vi "HFRR ADV v03.vi"() -> ()   [LabVIEW 2025] (continued)
                  n2418 = local write "S 85"(w3547) -> ()
                }
                frame 84 {
                  n2419 = local write "S 86"(w3548) -> ()
                }
                frame 85 {
                  n2420 = local write "S 87"(w3549) -> ()
                }
                frame 86 {
                  n2421 = local write "S 88"(w3550) -> ()
                }
                frame 87 {
                  n2422 = property on="FF Calibration g" class="WFGraph (strict)"("Y Scale.Name Label.Text"=w3551) -> ()  [unwired: 2 in, 2 out]
                }
                frame 88 {
                  n2423 = local write "S 90"(w3552) -> ()
                }
                frame 89 {
                  n2424 = local write "S 91"(w3553) -> ()
                }
                frame 90 {
                  n2425 = local write "S 92"(w3554) -> ()
                }
                frame 91 {
                  n2426 = local write "S 93"(w3555) -> ()
                }
                frame 92 {
                  n2427 = local write "S 94"(w3556) -> ()
                }
                frame 93 {
                  n2428 = local write "S 95"(w3557) -> ()
                }
                frame 94 {
                  n2429 = local write "S 96"(w3558) -> ()
                }
                frame 95 {
                  n2430 = local write "S 97"(w3559) -> ()
                }
                frame 96 {
                  n2431 = local write "S 98"(w3560) -> ()
                }
                frame 97 {
                  n2432 = local write "S 99"(w3561) -> ()
                }
                frame 98 {
                  n2433 = local write "S 100"(w3562) -> ()
                }
                frame 99 {
                  n2434 = local write "S 101"(w3563) -> ()
                }
                frame 100 {
                  n2435 = local write "S 102"(w3564) -> ()
                }
                frame 101 {
                  n2436 = local write "S 103"(w3565) -> ()
                }
                frame 102 {
                  n2437 = local write "S 104"(w3566) -> ()
                }
                frame 103 {
                  n2438 = local write "S 105"(w3567) -> ()
                }
                frame 104 {
                  n2439 = local write "S 106"(w3568) -> ()
                }
                frame 105 {
                }
                frame 106 {
                  n2440 = property on="OK Button 17" class="Bool (strict)"("Boolean Text.Text"=w3569) -> ()  [unwired: 2 in, 2 out]
                }
                frame 107 {
                  n2441 = property on="OK Button 16" class="Bool (strict)"("Boolean Text.Text"=w3570) -> ()  [unwired: 2 in, 2 out]
                }
                frame 108 {
                  n2442 = property on="TITTLE" class="Str"("Caption.Text"=w3571) -> ()  [unwired: 2 in, 2 out]
                }
                frame 109 {
                  "String 30" <- w3572
                }
                frame 110 {
                  n2443 = property on="Test Date" class="Str"("Caption.Text"=w3573) -> ()  [unwired: 2 in, 2 out]
                  "String 31" <- w3573
                }
                frame 111 {
                  n2444 = property on="Sample ID" class="Str"("Caption.Text"=w3574) -> ()  [unwired: 2 in, 2 out]
                  "String 32" <- w3574
                }
                frame 112 {
                  n2445 = property on="Tested by" class="Str"("Caption.Text"=w3575) -> ()  [unwired: 2 in, 2 out]
                  "String 33" <- w3575
                }
                frame 113 {
                  n2446 = property on="System Configured Printers 2" class="Arr (strict)"("Caption.Text"=w3576) -> ()  [unwired: 2 in, 2 out]
                }
                frame 114 {
                  n2447 = property on="Selected Printer" class="Str"("Caption.Text"=w3577) -> ()  [unwired: 2 in, 2 out]
                }
                frame 115 {
                  n2448 = property on="Select Printer 3" class="DigNum (strict)"("Caption.Text"=w3578) -> ()  [unwired: 2 in, 2 out]
                }
                frame 116 {
                  n2449 = property on="Print" class="Bool (strict)"("Boolean Text.Text"=w3579) -> ()  [unwired: 2 in, 2 out]
                }
                frame 117 {
                  "String 41" <- w3580
                }
                frame 118 {
                  n2450 = property on="tested by" class="Str"("Caption.Text"=w3581) -> ()  [unwired: 2 in, 2 out]
                }
                frame 119 {
                }
                frame 120 {
                  n2451 = property on="Export" class="Bool (strict)"("Boolean Text.Text"=w3582) -> ()  [unwired: 2 in, 2 out]
                }
                frame 121 {
                  n2452 = property on="TEMP INTERCEPT:" class="DigNum (strict)"("Caption.Text"=w3583) -> ()  [unwired: 2 in, 2 out]
                }
                frame 122 {
                  n2453 = property on="AIR TEMP INTERCEPT:" class="DigNum (strict)"("Caption.Text"=w3584) -> ()  [unwired: 2 in, 2 out]
                }
                frame 123 {
                  n2454 = property on="Select File Type" class="Enum (strict)"("Caption.Text"=w3585) -> ()  [unwired: 2 in, 2 out]
                }
                frame 124 {
                  n2455 = property on="s.NO" class="Str"("Caption.Text"=w3586) -> ()  [unwired: 2 in, 2 out]
                  "String 45" <- w3586
                }
                frame 125 {
                  n2456 = property on="trip1 8" class="Bool (strict)"("Boolean Text.Text"=w3587) -> ()  [unwired: 2 in, 2 out]
                }
                frame 126, Default {
                }
              }
            }
          }
          frame #1 {
            w3595 = TRUE ("Visible")
            n2457 = local read "S 91"() -> (w3612:string)
            n2458 = local read "S 90"() -> (w3611:string)
            n2459 = local read "S 88"() -> (w3610:string)
            n2460 = property on="Threshold" class="DigNum (strict)"("Caption.Text"=w3612) -> ()  [unwired: 2 in, 2 out]
            n2461 = property on="File Path" class="Path"("Caption.Text"=w3611) -> ()  [unwired: 2 in, 2 out]
            n2462 = property on="SrvM CP" class="Bool (strict)"("Boolean Text.Text"=w3610) -> ()  [unwired: 2 in, 2 out]
            n2463 = local read "S 71"() -> (w3605:string)
            n2464 = local read "S 86"() -> (w3607:string)
            n2465 = local read "S 85"() -> (w3608:string)
            n2466 = local read "S 87"() -> (w3606:string)
            n2467 = local read "S 84"() -> (w3609:string)
            n2468 = local read "S 103"() -> (w3594:string)
            n2469 = local read "S 104"() -> (w3593:string)
            n2470 = property on="ENTER THE NEW PASSWORD" class="Str"("Caption.Text"=w3606) -> ()  [unwired: 2 in, 2 out]
            n2471 = property on="Password" class="Str"("Caption.Text"=w3608) -> ()  [unwired: 2 in, 2 out]
            n2472 = property on="ENTER CURRENT PASSWORD" class="Str"("Caption.Text"=w3607) -> ()  [unwired: 2 in, 2 out]
            n2473 = property on="EDIT" class="Bool (strict)"("Boolean Text.Text"=w3605) -> ()  [unwired: 2 in, 2 out]
            n2474 = property on="SAVE" class="Bool (strict)"("Boolean Text.Text"=w3609) -> ()  [unwired: 2 in, 2 out]
            n2475 = Build Array(w3594, w3593) -> (w3592:string[])
            n2476 = property on="Heater Button" class="Bool (strict)"("Strings [4]"=w3592) -> ()  [unwired: 2 in, 2 out]
            n2477 = property on="CH-HUMIDITY WET" class="DigNum (strict)"("Caption.Size to Text?"=w3595) -> ()  [unwired: 2 in, 2 out]
            n2478 = property on="CH-HUMIDITY DRY" class="DigNum (strict)"("Caption.Size to Text?"=w3595) -> ()  [unwired: 2 in, 2 out]
            n2479 = property on="CH-POWER -" class="DigNum (strict)"("Caption.Size to Text?"=w3595) -> ()  [unwired: 2 in, 2 out]
            n2480 = property on="CH-HEATER" class="DigNum (strict)"("Caption.Size to Text?"=w3595) -> ()  [unwired: 2 in, 2 out]
            n2481 = property on="CH-POWER +" class="DigNum (strict)"("Caption.Size to Text?"=w3595) -> ()  [unwired: 2 in, 2 out]
            n2482 = local read "S 92"() -> (w3604:string)
            n2483 = local read "S 93"() -> (w3603:string)
            n2484 = local read "S 105"() -> (w3590:string)
            n2485 = local read "S 106"() -> (w3589:string)
            n2486 = Build Array(w3604, w3603) -> ()  [unwired: 1 out]
            n2487 = Build Array(w3590, w3589) -> (w3591:string[])
            n2488 = local read "S 95"() -> (w3601:string)
            n2489 = local read "S 94"() -> (w3602:string)
            n2490 = local read "bs"() -> (w3617:string)
            n2491 = local read "as"() -> (w3618:string)
            n2492 = property on="Humidity" class="Bool (strict)"("Strings [4]"=w3591) -> ()  [unwired: 2 in, 2 out]
            n2493 = Concatenate Strings(w3617, "\r", w3618) -> ()  [unwired: 1 out]
            n2494 = property on="STROKE GAIN :" class="DigNum (strict)"("Caption.Text"=w3601) -> ()  [unwired: 2 in, 2 out]
            n2495 = property on="DISPLACEMENT :" class="DigNum (strict)"("Caption.Text"=w3602) -> ()  [unwired: 2 in, 2 out]
            n2496 = property on="Rh After" class="DigNum (strict)"("Caption.Size to Text?"=TRUE ("Caption.Size to Text")) -> ()  [unwired: 2 in, 2 out]
            n2497 = local read "S 48"() -> (w3641:string)
            n2498 = local read "S 50"() -> (w3639:string)
            n2499 = local read "S 51"() -> (w3638:string)
            n2500 = local read "S 49"() -> (w3640:string)
            n2501 = local read "S 52"() -> (w3637:string)
            n2502 = local read "as"() -> (w3622:string)
            n2503 = local read "bs"() -> (w3623:string)
            n2504 = local read "S 56"() -> (w3636:string)
            n2505 = local read "S 57"() -> (w3635:string)
            n2506 = local read "S 58"() -> (w3634:string)
            n2507 = local read "S 59"() -> (w3633:string)
            n2508 = property on="OPEN" class="Bool (strict)"("Boolean Text.Text"=w3637) -> ()  [unwired: 2 in, 2 out]
            n2509 = property on="OPEN 1" class="Bool (strict)"("Boolean Text.Text"=w3641) -> ()  [unwired: 2 in, 2 out]
            n2510 = property on="OPEN 2" class="Bool (strict)"("Boolean Text.Text"=w3640) -> ()  [unwired: 2 in, 2 out]
            n2511 = property on="OPEN 3" class="Bool (strict)"("Boolean Text.Text"=w3639) -> ()  [unwired: 2 in, 2 out]
            n2512 = property on="OPEN 4" class="Bool (strict)"("Boolean Text.Text"=w3638) -> ()  [unwired: 2 in, 2 out]
            n2513 = Concatenate Strings(w3623, "\r", w3622) -> ()  [unwired: 1 out]
            n2514 = local read "S 102"() -> (w3596:string)
            n2515 = property on="КОФ1" class="DigNum (strict)"("Caption.Text"=w3636) -> ()  [unwired: 2 in, 2 out]
            n2516 = local read "S 98"() -> (w3600:string)
            n2517 = local read "S 99"() -> (w3599:string)
            n2518 = local read "S 100"() -> (w3598:string)
            n2519 = local read "S 101"() -> (w3597:string)
            n2520 = property on="КОФ2" class="DigNum (strict)"("Caption.Text"=w3635) -> ()  [unwired: 2 in, 2 out]
            n2521 = property on="КОФ3" class="DigNum (strict)"("Caption.Text"=w3634) -> ()  [unwired: 2 in, 2 out]
            n2522 = property on="КОФ4" class="DigNum (strict)"("Caption.Text"=w3633) -> ()  [unwired: 2 in, 2 out]
            n2523 = local read "bs"() -> (w3621:string)
            n2524 = local read "as"() -> (w3620:string)
            n2525 = property on="CH-POWER +" class="DigNum (strict)"("Caption.Text"=w3600) -> ()  [unwired: 2 in, 2 out]
            n2526 = property on="CH-POWER -" class="DigNum (strict)"("Caption.Text"=w3599) -> ()  [unwired: 2 in, 2 out]
            n2527 = property on="CH-HEATER" class="DigNum (strict)"("Caption.Text"=w3598) -> ()  [unwired: 2 in, 2 out]
            n2528 = property on="CH-HUMIDITY DRY" class="DigNum (strict)"("Caption.Text"=w3597) -> ()  [unwired: 2 in, 2 out]
            n2529 = property on="CH-HUMIDITY WET" class="DigNum (strict)"("Caption.Text"=w3596) -> ()  [unwired: 2 in, 2 out]
            n2530 = local read "S 60"() -> (w3632:string)
            n2531 = local read "S 54"() -> (w3642:string)
            n2532 = Concatenate Strings(w3621, "\r", w3620) -> ()  [unwired: 1 out]
            n2533 = Concatenate Strings(w3642, w3632) -> ()  [unwired: 1 out]
            n2534 = local read "S 77"() -> (→"String 43":string)
            n2535 = local read "S 76"() -> (w3615:string)
            n2536 = local read "S 78"() -> (w3614:string)
            n2537 = local read "S 71"() -> (w3626:string)
            n2538 = local read "S 66"() -> (w3631:string)
            n2539 = local read "S 67"() -> (w3630:string)
            n2540 = local read "S 68"() -> (w3629:string)
            n2541 = local read "S 69"() -> (w3628:string)
            n2542 = local read "S 70"() -> (w3627:string)
            n2543 = property on="AIR TEMP" class="DigNum (strict)"("Caption.Text"=w3614) -> ()  [unwired: 2 in, 2 out]
            n2544 = property on="Set Strk" class="DigNum (strict)"("Caption.Text"=w3615) -> ()  [unwired: 2 in, 2 out]
            n2545 = property on="FRIC. FORCE :" class="DigNum (strict)"("Caption.Text"=w3631) -> ()  [unwired: 2 in, 2 out]
            n2546 = property on="TEMPERATURE :" class="DigNum (strict)"("Caption.Text"=w3630) -> ()  [unwired: 2 in, 2 out]
            n2547 = property on="SPEED OUT:" class="DigNum (strict)"("Caption.Text"=w3629) -> ()  [unwired: 2 in, 2 out]
            n2548 = property on="AIR TEMPERATURE :" class="DigNum (strict)"("Caption.Text"=w3628) -> ()  [unwired: 2 in, 2 out]
            n2549 = property on="HUMIDITY:" class="DigNum (strict)"("Caption.Text"=w3627) -> ()  [unwired: 2 in, 2 out]
            n2550 = property on="EDIT" class="Bool (strict)"("Boolean Text.Text"=w3626) -> ()  [unwired: 2 in, 2 out]
            n2551 = local read "S 79"() -> (w3613:string)
            n2552 = property on="Stroke" class="DigNum (strict)"("Caption.Text"=w3613) -> ()  [unwired: 2 in, 2 out]
          }
          frame #2 {
          }
        }
        n2553 = local write "Lan flag"(10.0 ("Lan flag")) -> ()
      }
    }
    n2554 = Wait (ms)(milliseconds to wait=u32 50) -> ()  [unwired: 1 out]
    n2555 = local read "EXIT"() -> (w3418:bool)
  }
  n2556 = flat-sequence {
    tunnel: w50 -> [_]
    frame #0 {
    }
    frame #1 {
      n2557 = Quit LabVIEW(quit? (T)=TRUE) -> ()
      n2558 = local write "EXIT"(FALSE ("EXIT")) -> ()
    }
  }
  n2559 = while {
    tunnel: [w3652] -> w48
    i -> [w3651]
    stop <- w3652 stop-if-true
    n2560 = local read "EXIT"() -> (w3652:bool)
    n2561 = Equal To 0?(x=w3651) -> (x = 0?=w3649:bool)
    n2562 = call "Elapsed Time3"("Time Target (s)"=45.0, "Auto Reset"=TRUE) -> ("Time has Elapsed"=w3648:bool)  [unwired: 10 in, 7 out]
    n2563 = Wait (ms)(milliseconds to wait=u32 50) -> ()  [unwired: 1 out]
    n2564 = Or(x=w3648, y=w3649) -> (x .or. y?=w3650:bool)
    n2565 = case shown="True" w3650 {
      frame False {
      }
      frame True {
        n2566 = call <vilib>:"System Exec.vi"("run minimized? (F)"=TRUE, "error in (no error)"="error in (no error)", "command line"="powercfg.exe -change -monitor-timeout-ac 0") -> ("error out"=w3663:errorcluster)  [unwired: 5 in, 3 out]
        n2567 = call <vilib>:"System Exec.vi"("run minimized? (F)"=TRUE, "error in (no error)"=w3663, "command line"="powercfg.exe -change -disk-timeout-ac 0") -> ("error out"=w3662:errorcluster)  [unwired: 5 in, 3 out]
        n2568 = call <vilib>:"System Exec.vi"("run minimized? (F)"=TRUE, "error in (no error)"=w3662, "command line"="powercfg.exe -change -standby-timeout-ac 0") -> ("error out"=w3661:errorcluster)  [unwired: 5 in, 3 out]
        n2569 = call <vilib>:"System Exec.vi"("run minimized? (F)"=TRUE, "error in (no error)"=w3661, "command line"="powercfg.exe -change -hibernate-timeout-ac 0") -> ("error out"=w3660:errorcluster)  [unwired: 5 in, 3 out]
        n2570 = call <vilib>:"Simple Error Handler.vi"("error in (no error)"=w3660) -> ("error out"=w3666:errorcluster)  [unwired: 4 in, 4 out]
        n2571 = call <vilib>:"Clear Errors.vi"("error in (no error)"=w3666) -> ("error out"=→"error out":errorcluster)  [unwired: 5 in, 1 out]
      }
    }
  }
  n2572 = Compound Arithmetic op=OR(w51, w52, w48) -> (w50:bool)
  n2573 = while {
    shift-right: [w3673] -> _
    shift-left: _ -> [w3674]
    shift-right: [w3671] -> _
    shift-left: T10 {"Read Heave and Surge"="", "Bytes at Heave Port"=0.0, "Heave and Surge COM Port:"="COM9", "Com Port 2"="COM7", "Residual Due"="", "Heave COM Status 2"=TRUE, "Heave COM Status"=TRUE, "Port 2"=TRUE, "Sway PPR"=6400.0, "Surge PPR"=6400.0, "Heave PPR"=6400.0, "Sway Pitch"=2.0, "Surge Pitch"=3.0, "Heave Pitch"=4.0, "Sway Pulses/mm"=320.0, "Surge Pulses/mm"=1600.0, "Heave Pulses/mm"=1600.0, "inner loop"=0.0, "Read Heave and Surge 2"="", "String 36"="", "Write S"=FALSE, "WriteCC1"=[""], "Heave COM Loop"=0, "LastCom"="", "EXIT"=FALSE, "Error Heave"={"status"=TRUE, "code"=-1073807343, "source"=""}} -> [w3670]
    shift-right: [w3668] -> _
    shift-left: enum16{"init", "MAIN", "Panel Close"}."init" -> [w3669]
    stop <- w3672 stop-if-true
    n2574 = case shown="\"MAIN\"" w3669 {
      tunnel: w3674 -> [w3688 w3703 w3773 w3775]
      tunnel: [w3682 w3721 w3773 w3775] -> w3673
      tunnel: [_ _ TRUE _] -> w3672
      tunnel: [w3678 w3718 w3771 w3774] -> w3671
      tunnel: w3670 -> [w3685 w3702 w3771 w3774]
      tunnel: [enum16{"init", "MAIN", "Panel Close"}."MAIN" w3696 _ _] -> w3668
      frame "init" {
        n2575 = Bundle By Name(cluster=w3685, "Heave and Surge COM Port:"="Instrument Com Port") -> (w3684:T10)
        n2576 = call "Instrument fgv.vi"("Enum"=T18."INIT", "error in (no error) 2"=w3688, "INPUT"=w3684) -> ("error"=w3686:errorcluster, "output"=w3681:T10)  [unwired: 6 in, 1 out]
        n2577 = case shown="Error" w3686 {
          selector: w3686 -> [w3690 _]
          tunnel: [w3690 w3694] -> w3682
          tunnel: w3681 -> [w3689 w3692]
          tunnel: [w3689 w3691] -> w3679
          frame No Error {
          }
          frame Error {
            n2578 = call "Instrument fgv.vi"("Enum"=T18."ERROR INIT", "INPUT"=w3692) -> ("error"=w3695:errorcluster, "output"=w3691:T10)  [unwired: 7 in, 1 out]
            n2579 = call <vilib>:"Clear Errors.vi"("error in (no error)"=w3695) -> ("error out"=w3694:errorcluster)  [unwired: 5 in, 1 out]
          }
        }
        n2580 = local read "LastCom"() -> (w3677:string)
        n2581 = Unbundle By Name(w3679) -> ("Heave COM Status 2"=→"Heave COM Status 2" →"Instrument Status":bool, "Error Heave"=→"Error Heave":errorcluster)  [unwired: 1 out]
        n2582 = Bundle By Name(cluster=w3679, "LastCom"=w3677) -> (w3678:T10)
      }
      frame "MAIN" {
        n2583 = Unbundle By Name(w3702) -> ("Com Port 2"=w3723:refnum<visa-resource-name>)
        n2584 = local read "Instrument Com Port"() -> (w3700:refnum<visa-resource-name>)
        n2585 = local write "Com Port 4"(w3723) -> ()
        n2586 = Divide(x="Heave PPR", y="Heave Pitch") -> (x/y=→"Heave Pulses/mm":dbl)
        n2587 = Bundle By Name(cluster=w3702, "Heave and Surge COM Port:"=w3700) -> (w3701:T10)
        n2588 = Equal?(x=w3723, y=w3700) -> (x = y?=w3722:bool)
        n2589 = Divide(x="Sway PPR", y="Sway Pitch") -> (x/y=→"Sway Pulses/mm":dbl)
        n2590 = Divide(x="Surge PPR", y="Surge Pitch") -> (x/y=→"Surge Pulses/mm":dbl)
        n2591 = case shown="True" w3722 {
          tunnel: [w3727 w3744] -> w3721
          tunnel: w3703 -> [w3728 w3750]
          tunnel: w3701 -> [w3726 w3748]
          tunnel: [w3725 w3743] -> w3718
          frame False {
            n2592 = call <vilib>:"Clear Errors.vi"("error in (no error)"=w3728) -> ("error out"=w3724:errorcluster)  [unwired: 5 in, 1 out]
            n2593 = call "Instrument fgv.vi"("Enum"=T18."ERROR INIT", "error in (no error) 2"=w3724, "INPUT"=w3726) -> ("error"=w3730:errorcluster, "output"=w3725:T10)  [unwired: 6 in, 1 out]
            n2594 = call <vilib>:"Clear Errors.vi"("error in (no error)"=w3730) -> ("error out"=w3727:errorcluster)  [unwired: 5 in, 1 out]
          }
          frame True {
            n2595 = call "Instrument fgv.vi"("Enum"=T18."READ", "error in (no error) 2"=w3750, "INPUT"=w3748) -> ("error"=w3749:errorcluster, "output"=w3740:T10)  [unwired: 6 in, 1 out]
            n2596 = Bundle By Name(cluster=w3740, "String 36"="String") -> (w3739:T10)
            n2597 = case shown="True" "Write S" {
              selector: "Write S" -> [_ w3770]
              tunnel: w3749 -> [w3763 w3769]
              tunnel: [w3763 w3768] -> w3736
              tunnel: w3739 -> [w3762 w3765]
              tunnel: [w3762 w3764] -> w3735
              frame False {
              }
              frame True {
                n2598 = Not(x=w3770) -> (.not. x?=w3766:bool)
                n2599 = local write "Write S"(w3766) -> ()
                n2600 = call "Instrument fgv.vi"("Enum"=T18."MANUAL WRITE", "error in (no error) 2"=w3769, "INPUT"=w3765) -> ("error"=w3768:errorcluster, "output"=w3764:T10)  [unwired: 6 in, 1 out]
              }
            }
            n2601 = Array Size(array="WriteCC1") -> (size(s)=w3733:i32)
            n2602 = Greater Than 0?(x=w3733) -> (x > 0?=w3731:bool)
            n2603 = call "Instrument fgv.vi"("Enum"=T18."WRITE", "error in (no error) 2"=w3736, "WriteCC1"="WriteCC1", "INPUT"=w3735) -> ("error"=w3746:errorcluster, "WriteCC1 2"=w3734:string[], "output"=w3745:T10)  [unwired: 5 in]
            n2604 = case shown="True" w3731 {
              tunnel: w3734 -> [_ w3752]
              frame False {
              }
              frame True {
                n2605 = local write "WriteCC1"(w3752) -> ()
              }
            }
            n2606 = case shown="Error" w3746 {
              selector: w3746 -> [w3753 w3756]
              tunnel: w3745 -> [w3754 w3761]
              tunnel: [w3754 w3760] -> w3743
              tunnel: [w3753 w3758] -> w3744
              frame No Error {
              }
              frame Error {
                n2607 = call <vilib>:"Clear Errors.vi"("error in (no error)"=w3756) -> ("error out"=w3755:errorcluster)  [unwired: 5 in, 1 out]
                n2608 = call "Instrument fgv.vi"("Enum"=T18."ERROR INIT", "error in (no error) 2"=w3755, "INPUT"=w3761) -> ("error"=w3759:errorcluster, "output"=w3760:T10)  [unwired: 6 in, 1 out]
                n2609 = call <vilib>:"Clear Errors.vi"("error in (no error)"=w3759) -> ("error out"=w3758:errorcluster)  [unwired: 5 in, 1 out]
              }
            }
            n2610 = Unbundle By Name(w3743) -> ("LastCom"=→"LastCom":string, "Read Heave and Surge"=→"Read Humidity":string)
          }
        }
        n2611 = Unbundle By Name(w3718) -> ("Heave COM Status 2"=w3720:bool, "Heave COM Status"=w3719:bool, "Error Heave"=w3716:errorcluster, "Bytes at Heave Port"=→"Bytes at Humidity Port":dbl)
        n2612 = local read "Quit"() -> (w3697:bool)
        n2613 = local write "Error Heave"(w3716) -> ()
        n2614 = Unbundle By Name(w3716) -> ("status"=→"Port 5":bool)
        n2615 = Not(x=w3719) -> (.not. x?=w3704:bool)
        n2616 = Not(x=w3720) -> (.not. x?=w3705:bool)
        n2617 = local write "Instrument Status"(w3704) -> ()
        n2618 = local write "Heave COM Status 2"(w3705) -> ()
        n2619 = Select(t=enum16{"init", "MAIN", "Panel Close"}."Panel Close", s=w3697, f=enum16{"init", "MAIN", "Panel Close"}."MAIN") -> (s? t:f=w3696:enum16{"init", "MAIN", "Panel Close"})
      }
      frame "Panel Close" {
      }
      frame Default {
      }
    }
  }
  n2620 = case shown="True" "Case Constant\n(See Context Help) 6" {
    tunnel: w23 -> [_ w3776]
    frame False {
    }
    frame True {
      n2621 = while {
        tunnel: w3776 -> [_]
        tunnel: [w3777] -> _
        i -> [w3777]
        stop <- w3778 continue-if-true
        n2622 = Wait (ms)(milliseconds to wait=u32 50) -> ()  [unwired: 1 out]
        n2623 = stacked-sequence {
          frame #0 {
            # "Controls Text color"
            # "Controls BG color"
            n2624 = property on="FILE" class="Str"("Text.Text Colors:Text Color"="SC  Text") -> ()  [unwired: 2 in, 2 out]
            n2625 = property on="Fuel Discription :" class="Str"("Text.Text Colors:Text Color"="SC  Text") -> ()  [unwired: 2 in, 2 out]
            n2626 = property on="tested by" class="Str"("Text.Text Colors:Text Color"="SC  Text") -> ()  [unwired: 2 in, 2 out]
            n2627 = property on="Remarks :" class="Str"("Text.Text Colors:Text Color"="SC  Text") -> ()  [unwired: 2 in, 2 out]
            n2628 = property class="DigNum (strict)"("Numeric Text.Text Colors:BG Color"="NC BG") -> ()  [unwired: 2 in, 2 out]
            n2629 = property class="DigNum (strict)"("Numeric Text.Text Colors:BG Color"="NC BG") -> ()  [unwired: 2 in, 2 out]
            n2630 = property class="DigNum (strict)"("Numeric Text.Text Colors:BG Color"="NC BG") -> ()  [unwired: 2 in, 2 out]
            n2631 = property class="DigNum (strict)"("Numeric Text.Text Colors:BG Color"="NC BG") -> ()  [unwired: 2 in, 2 out]
            n2632 = property class="DigNum (strict)"("Numeric Text.Text Colors:BG Color"="NC BG") -> ()  [unwired: 2 in, 2 out]
            n2633 = property class="DigNum (strict)"("Numeric Text.Text Colors:BG Color"="NC BG") -> ()  [unwired: 2 in, 2 out]
            n2634 = property class="DigNum (strict)"("Numeric Text.Text Colors:BG Color"="NC BG") -> ()  [unwired: 2 in, 2 out]
            n2635 = property class="DigNum (strict)"("Numeric Text.Text Colors:BG Color"="NC BG") -> ()  [unwired: 2 in, 2 out]
            n2636 = property class="DigNum (strict)"("Numeric Text.Text Colors:BG Color"="NC BG") -> ()  [unwired: 2 in, 2 out]
            n2637 = property class="DigNum (strict)"("Numeric Text.Text Colors:BG Color"="NC BG") -> ()  [unwired: 2 in, 2 out]
            n2638 = property class="DigNum (strict)"("Numeric Text.Text Colors:BG Color"="NC BG") -> ()  [unwired: 2 in, 2 out]
            n2639 = property class="DigNum (strict)"("Numeric Text.Text Colors:BG Color"="NC BG") -> ()  [unwired: 2 in, 2 out]
            n2640 = property on="FILE" class="Str"("Text.Text Colors:BG Color"="SC BG 3") -> ()  [unwired: 2 in, 2 out]
            n2641 = property on="Fuel Discription :" class="Str"("Text.Text Colors:BG Color"="SC BG 3") -> ()  [unwired: 2 in, 2 out]
            n2642 = property on="tested by" class="Str"("Text.Text Colors:BG Color"="SC BG 3") -> ()  [unwired: 2 in, 2 out]
            n2643 = property on="Remarks :" class="Str"("Text.Text Colors:BG Color"="SC BG 3") -> ()  [unwired: 2 in, 2 out]
            n2644 = property class="DigNum (strict)"("Numeric Text.Text Colors:Text Color"="NC Text") -> ()  [unwired: 2 in, 2 out]
            n2645 = property class="DigNum (strict)"("Numeric Text.Text Colors:Text Color"="NC Text") -> ()  [unwired: 2 in, 2 out]
            n2646 = property class="DigNum (strict)"("Numeric Text.Text Colors:Text Color"="NC Text") -> ()  [unwired: 2 in, 2 out]
            n2647 = property class="DigNum (strict)"("Numeric Text.Text Colors:Text Color"="NC Text") -> ()  [unwired: 2 in, 2 out]
            n2648 = property class="DigNum (strict)"("Numeric Text.Text Colors:Text Color"="NC Text") -> ()  [unwired: 2 in, 2 out]
            n2649 = property class="DigNum (strict)"("Numeric Text.Text Colors:Text Color"="NC Text") -> ()  [unwired: 2 in, 2 out]
            n2650 = property class="DigNum (strict)"("Numeric Text.Text Colors:Text Color"="NC Text") -> ()  [unwired: 2 in, 2 out]
            n2651 = property class="DigNum (strict)"("Numeric Text.Text Colors:Text Color"="NC Text") -> ()  [unwired: 2 in, 2 out]
            n2652 = property class="DigNum (strict)"("Numeric Text.Text Colors:Text Color"="NC Text") -> ()  [unwired: 2 in, 2 out]
            n2653 = property class="DigNum (strict)"("Numeric Text.Text Colors:Text Color"="NC Text") -> ()  [unwired: 2 in, 2 out]
            n2654 = property class="DigNum (strict)"("Numeric Text.Text Colors:Text Color"="NC Text") -> ()  [unwired: 2 in, 2 out]
            n2655 = property class="DigNum (strict)"("Numeric Text.Text Colors:Text Color"="NC Text") -> ()  [unwired: 2 in, 2 out]
            n2656 = property class="DigNum (strict)"("Numeric Text.Text Colors:Text Color"="NI Text  2") -> ()  [unwired: 2 in, 2 out]
            n2657 = property class="DigNum (strict)"("Numeric Text.Text Colors:Text Color"="NI Text  2") -> ()  [unwired: 2 in, 2 out]
            n2658 = property class="DigNum (strict)"("Numeric Text.Text Colors:Text Color"="NI Text  2") -> ()  [unwired: 2 in, 2 out]
            n2659 = property class="DigNum (strict)"("Numeric Text.Text Colors:Text Color"="NI Text  2") -> ()  [unwired: 2 in, 2 out]
            n2660 = property class="DigNum (strict)"("Numeric Text.Text Colors:Text Color"="NI Text  2") -> ()  [unwired: 2 in, 2 out]
            n2661 = property class="DigNum (strict)"("Numeric Text.Text Colors:Text Color"="NI Text  2") -> ()  [unwired: 2 in, 2 out]
            n2662 = property class="DigNum (strict)"("Numeric Text.Text Colors:Text Color"="NI Text  2") -> ()  [unwired: 2 in, 2 out]
            n2663 = property class="DigNum (strict)"("Numeric Text.Text Colors:Text Color"="NI Text  2") -> ()  [unwired: 2 in, 2 out]
            n2664 = property class="DigNum (strict)"("Numeric Text.Text Colors:Text Color"="NI Text  2") -> ()  [unwired: 2 in, 2 out]
            n2665 = property class="DigNum (strict)"("Numeric Text.Text Colors:Text Color"="NI Text  2") -> ()  [unwired: 2 in, 2 out]
            n2666 = property class="DigNum (strict)"("Numeric Text.Text Colors:Text Color"="NI Text  2") -> ()  [unwired: 2 in, 2 out]
            n2667 = property class="DigNum (strict)"("Numeric Text.Text Colors:Text Color"="NI Text  2") -> ()  [unwired: 2 in, 2 out]
            n2668 = property class="DigNum (strict)"("Numeric Text.Text Colors:Text Color"="NI Text  2") -> ()  [unwired: 2 in, 2 out]
            n2669 = property class="DigNum (strict)"("Numeric Text.Text Colors:Text Color"="NI Text  2") -> ()  [unwired: 2 in, 2 out]
            n2670 = property class="DigNum (strict)"("Numeric Text.Text Colors:Text Color"="NI Text  2") -> ()  [unwired: 2 in, 2 out]
            n2671 = property class="DigNum (strict)"("Numeric Text.Text Colors:Text Color"="NI Text  2") -> ()  [unwired: 2 in, 2 out]
            n2672 = property on="Coefficient Of Friction" class="XYGraph (strict)"("Plot Area:Colors:FG Color"="GFG  2", "Plot Area:Colors:BG Color"="GBG   2") -> ()  [unwired: 2 in, 2 out]
            n2673 = property on="Humidity" class="XYGraph (strict)"("Plot Area:Colors:FG Color"="GFG  2", "Plot Area:Colors:BG Color"="GBG   2") -> ()  [unwired: 2 in, 2 out]
            n2674 = property on="Air Temperature" class="XYGraph (strict)"("Plot Area:Colors:FG Color"="GFG  2", "Plot Area:Colors:BG Color"="GBG   2") -> ()  [unwired: 2 in, 2 out]
            n2675 = property on="Sample Temperature" class="XYGraph (strict)"("Plot Area:Colors:FG Color"="GFG  2", "Plot Area:Colors:BG Color"="GBG   2") -> ()  [unwired: 2 in, 2 out]
            n2676 = property class="DigNum (strict)"("Numeric Text.Text Colors:BG Color"="NI BG 2") -> ()  [unwired: 2 in, 2 out]
            n2677 = property class="DigNum (strict)"("Numeric Text.Text Colors:BG Color"="NI BG 2") -> ()  [unwired: 2 in, 2 out]
            n2678 = property class="DigNum (strict)"("Numeric Text.Text Colors:BG Color"="NI BG 2") -> ()  [unwired: 2 in, 2 out]
            n2679 = property class="DigNum (strict)"("Numeric Text.Text Colors:BG Color"="NI BG 2") -> ()  [unwired: 2 in, 2 out]
            n2680 = property class="DigNum (strict)"("Numeric Text.Text Colors:BG Color"="NI BG 2") -> ()  [unwired: 2 in, 2 out]
            n2681 = property class="DigNum (strict)"("Numeric Text.Text Colors:BG Color"="NI BG 2") -> ()  [unwired: 2 in, 2 out]
            n2682 = property class="DigNum (strict)"("Numeric Text.Text Colors:BG Color"="NI BG 2") -> ()  [unwired: 2 in, 2 out]
            n2683 = property class="DigNum (strict)"("Numeric Text.Text Colors:BG Color"="NI BG 2") -> ()  [unwired: 2 in, 2 out]
            n2684 = property class="DigNum (strict)"("Numeric Text.Text Colors:BG Color"="NI BG 2") -> ()  [unwired: 2 in, 2 out]
            n2685 = property class="DigNum (strict)"("Numeric Text.Text Colors:BG Color"="NI BG 2") -> ()  [unwired: 2 in, 2 out]
            n2686 = property class="DigNum (strict)"("Numeric Text.Text Colors:BG Color"="NI BG 2") -> ()  [unwired: 2 in, 2 out]
            n2687 = property class="DigNum (strict)"("Numeric Text.Text Colors:BG Color"="NI BG 2") -> ()  [unwired: 2 in, 2 out]
            n2688 = property class="DigNum (strict)"("Numeric Text.Text Colors:BG Color"="NI BG 2") -> ()  [unwired: 2 in, 2 out]
            n2689 = property class="DigNum (strict)"("Numeric Text.Text Colors:BG Color"="NI BG 2") -> ()  [unwired: 2 in, 2 out]
            n2690 = property class="DigNum (strict)"("Numeric Text.Text Colors:BG Color"="NI BG 2") -> ()  [unwired: 2 in, 2 out]
            n2691 = property class="DigNum (strict)"("Numeric Text.Text Colors:BG Color"="NI BG 2") -> ()  [unwired: 2 in, 2 out]
            n2692 = property class="Bool"("Colors [4]"="Boolean BC T & BG") -> ()  [unwired: 2 in, 2 out]
            n2693 = property on="Save & Continue" class="Bool (strict)"("Colors [4]"="Boolean BC T & BG") -> ()  [unwired: 2 in, 2 out]
            n2694 = property on="STOP 3" class="Bool (strict)"("Colors [4]"="Boolean BC T & BG") -> ()  [unwired: 2 in, 2 out]
            n2695 = property on="Heater Button" class="Bool (strict)"("Colors [4]"="Boolean BC T & BG") -> ()  [unwired: 2 in, 2 out]
            n2696 = property class="Bool"("Colors [4]"="Boolean BC T & BG") -> ()  [unwired: 2 in, 2 out]
            n2697 = property on="Humidity" class="Bool (strict)"("Colors [4]"="Boolean BC T & BG") -> ()  [unwired: 2 in, 2 out]
            n2698 = property class="Bool (strict)"("Colors [4]"="Boolean BC T & BG") -> ()  [unwired: 2 in, 2 out]
            n2699 = property on="RUN" class="Bool (strict)"("Colors [4]"="Boolean BC T & BG") -> ()  [unwired: 2 in, 2 out]
            n2700 = property on="trip1 8" class="Bool (strict)"("Colors [4]"="Boolean BC T & BG") -> ()  [unwired: 2 in, 2 out]
            n2701 = property class="Bool"("Colors [4]"="Boolean BC T & BG") -> ()  [unwired: 2 in, 2 out]
            n2702 = property class="Bool (strict)"("Colors [4]"="Boolean BC T & BG") -> ()  [unwired: 2 in, 2 out]
            n2703 = property on="OPEN 1" class="Bool (strict)"("Colors [4]"="Boolean BC T & BG 2") -> ()  [unwired: 2 in, 2 out]
            n2704 = property on="OPEN 2" class="Bool (strict)"("Colors [4]"="Boolean BC T & BG 2") -> ()  [unwired: 2 in, 2 out]
            n2705 = property on="OPEN 3" class="Bool (strict)"("Colors [4]"="Boolean BC T & BG 2") -> ()  [unwired: 2 in, 2 out]
            n2706 = property on="OPEN 4" class="Bool (strict)"("Colors [4]"="Boolean BC T & BG 2") -> ()  [unwired: 2 in, 2 out]
            n2707 = property on="OPEN" class="Bool (strict)"("Colors [4]"="Boolean BC T & BG 2") -> ()  [unwired: 2 in, 2 out]
            n2708 = property on="rstv2" class="Bool"("Colors [4]"="Boolean BC T & BG 2") -> ()  [unwired: 2 in, 2 out]
            n2709 = property on="RST CP" class="Bool"("Colors [4]"="Boolean BC T & BG 2") -> ()  [unwired: 2 in, 2 out]
            n2710 = property on="RSTV1 3" class="Bool"("Colors [4]"="Boolean BC T & BG 2") -> ()  [unwired: 2 in, 2 out]
            n2711 = property on="RSTV1 2" class="Bool"("Colors [4]"="Boolean BC T & BG 2") -> ()  [unwired: 2 in, 2 out]
          }
          frame #1 {
          }
        }
        n2712 = local read "EXIT"() -> (w3778:bool)
      }
    }
  }
  n2713 = case shown="True" "Case Constant\n(See Context Help)" {
    frame False {
    }
    frame True {
      n2714 = while {
        tunnel: [w4026] -> _
        i -> [w4026]
        stop <- w4024 stop-if-true
        n2715 = local read "powstat"() -> (w4023:bool)
        n2716 = case shown="True" w4023 {
          frame False {
          }
          frame True {
            n2717 = local read "RUN"() -> (w4027:bool)
            n2718 = case shown="True" w4027 {
              frame False {
                w4057 = 65.0 ("y")
                n2719 = local read "Set Hz"() -> (w4085:dbl)
                n2720 = local read "NORMAL LOAD"() -> (w4086:dbl)
                n2721 = Multiply(x=w4085, y=60.0) -> (x*y=w4092:dbl)
                n2722 = Multiply(x=1.2 ("y"), y=0.949) -> (x*y=w4061:dbl)
                n2723 = Multiply(x=1.2 ("y"), y=0.8166) -> (x*y=w4065:dbl)
                n2724 = Multiply(x=1.2 ("y"), y=0.851) -> (x*y=w4060:dbl)
                n2725 = local read "FF 2"() -> (w4084:dbl)
                n2726 = Absolute Value(x=w4092) -> (abs(x)=w4090:dbl)
                n2727 = local read "Stroke"() -> (w4059:dbl)
                n2728 = Less?(x=w4059, y=w4065) -> (x < y?=w4062:bool)
                n2729 = In Range and Coerce(upper limit=w4061, x=w4059, lower limit=w4060) -> (In Range?=w4063:bool)  [unwired: 1 out]
                n2730 = case shown="13.." w4084 {
                  tunnel: [1 2 3] -> w4082
                  frame 0..10, Default {
                    # "Normal"
                  }
                  frame 11, 12 {
                  }
                  frame 13.. {
                  }
                }
                "FF STATE" <- w4082
                n2731 = local read "TEMP"() -> (w4045:dbl)
                n2732 = case shown="3601.." w4090 {
                  tunnel: [1 2 3] -> w4088
                  frame 0..3000, Default {
                    # "Normal"
                  }
                  frame 3001..3600 {
                  }
                  frame 3601.. {
                  }
                }
                n2733 = case shown="11.." w4086 {
                  tunnel: [1 3] -> w4087
                  frame 1..10, Default {
                  }
                  frame 11.. {
                  }
                }
                "NL STATE" <- w4087
                n2734 = Multiply(x=1.2 ("y"), y=0.95) -> (x*y=w4075:dbl)
                n2735 = Multiply(x=w4057, y=0.954) -> (x*y=w4049:dbl)
                n2736 = Or(x=w4062, y=w4063) -> (x .or. y?=w4064:bool)
                n2737 = Greater Or Equal?(x=w4059, y=w4075) -> (x >= y?=w4072:bool)
                n2738 = Multiply(x=w4057, y=0.99) -> (x*y=w4046:dbl)
                n2739 = Greater Or Equal?(x=w4045, y=w4046) -> (x >= y?=w4051:bool)
                n2740 = Greater Or Equal?(x=w4045, y=w4049) -> (x >= y?=w4048:bool)
                n2741 = case shown="0, 1, Default" w4059 {
                  tunnel: [1 3] -> w4076
                  frame 0, 1, Default {
                  }
                  frame 2.. {
                  }
                }
                n2742 = case shown="True" w4072 {
                  tunnel: [1 3] -> w4077
                  frame False {
                  }
                  frame True {
                  }
                }
                n2743 = case shown="True" w4064 {
                  tunnel: [1 2] -> w4078
                  frame False {
                  }
                  frame True {
                  }
                }
                n2744 = case shown="..0" w4045 {
                  tunnel: [2 3 3 1] -> w4052
                  frame 61, 62 {
                  }
                  frame 63.. {
                  }
                  frame ..0 {
                  }
                  frame 10..60, Default {
                  }
                }
                n2745 = case shown="True" w4051 {
                  tunnel: [1 3] -> w4053
                  frame False {
                  }
                  frame True {
                  }
                }
                n2746 = Number To Decimal String(number=w4088) -> (decimal integer string=w4089:string)  [unwired: 1 in]
                n2747 = case shown="True" w4048 {
                  tunnel: [1 2] -> w4054
                  frame False {
                  }
                  frame True {
                  }
                }
                n2748 = Number To Decimal String(number=1) -> (decimal integer string=→"Air temp":string)  [unwired: 1 in]
                n2749 = Number To Decimal String(number=w4082) -> (decimal integer string=→"ff_st":string)  [unwired: 1 in]
                n2750 = local write "sp_st"(w4089) -> ()
                n2751 = Number To Decimal String(number=w4087) -> (decimal integer string=→"nl_st":string)  [unwired: 1 in]
                n2752 = Build Array(w4052, w4053, w4054) -> (w4055:i32[])
                n2753 = Build Array(w4076, w4077, w4078) -> (w4079:i32[])
                n2754 = Array Max & Min(array=w4055) -> (max value=w4056:i32)  [unwired: 3 out]
                n2755 = Array Max & Min(array=w4079) -> (max value=w4080:i32)  [unwired: 3 out]
                n2756 = Number To Decimal String(number=w4056) -> (decimal integer string=w4044:string)  [unwired: 1 in]
                n2757 = Number To Decimal String(number=w4080) -> (decimal integer string=→"Stroke Ln 2":string)  [unwired: 1 in]
                n2758 = local write "temp_st"(w4044) -> ()
              }
              frame True {
                w4142 = 65.0 ("y")
                # "Healthy -1\nWarning -2\nError -3"
                n2759 = local read "TEMP"() -> (w4153:dbl)
                n2760 = local read "NORMAL LOAD"() -> (w4157:dbl)
                n2761 = local read "Set Hz"() -> (w4155:dbl)
                n2762 = Multiply(x=1.2 ("y"), y=0.949) -> (x*y=w4137:dbl)
                n2763 = Multiply(x=1.2 ("y"), y=0.8166) -> (x*y=w4133:dbl)
                n2764 = Multiply(x=1.2 ("y"), y=0.851) -> (x*y=w4138:dbl)
                n2765 = Multiply(x=w4142, y=0.954) -> (x*y=w4149:dbl)
                n2766 = Multiply(x=w4142, y=0.99) -> (x*y=w4152:dbl)
                n2767 = Greater Or Equal?(x=w4153, y=w4152) -> (x >= y?=w4147:bool)
                n2768 = Multiply(x=w4155, y=60.0) -> (x*y=w4161:dbl)
                n2769 = Greater Or Equal?(x=w4153, y=w4149) -> (x >= y?=w4150:bool)
                n2770 = local read "FF 2"() -> (w4156:dbl)
                n2771 = local read "Stroke"() -> (w4139:dbl)
                n2772 = Less?(x=w4139, y=w4133) -> (x < y?=w4136:bool)
                n2773 = In Range and Coerce(upper limit=w4137, x=w4139, lower limit=w4138) -> (In Range?=w4135:bool)  [unwired: 1 out]
                n2774 = Absolute Value(x=w4161) -> (abs(x)=w4159:dbl)
                n2775 = case shown="63.." w4153 {
                  tunnel: [2 3 3 1] -> w4146
                  frame 61, 62 {
                  }
                  frame 63.. {
                  }
                  frame ..0 {
                  }
                  frame 10..60, Default {
                  }
                }
                n2776 = case shown="True" w4147 {
                  tunnel: [1 3] -> w4145
                  frame False {
                  }
                  frame True {
                  }
                }
                n2777 = case shown="True" w4150 {
                  tunnel: [1 2] -> w4144
                  frame False {
                  }
                  frame True {
                  }
                }
                n2778 = Multiply(x=1.2 ("y"), y=0.95) -> (x*y=w4123:dbl)
                n2779 = case shown="1..10, Default" w4157 {
                  tunnel: [1 3] -> w4164
                  frame 1..10, Default {
                  }
                  frame 11.. {
                  }
                }
                n2780 = case shown="0..10, Default" w4156 {
                  tunnel: [1 2 3] -> w4163
                  frame 0..10, Default {
                  }
                  frame 11, 12 {
                  }
                  frame 13.. {
                  }
                }
                n2781 = case shown="3601.." w4159 {
                  tunnel: [1 2 3] -> w4158
                  frame 0..3000, Default {
                    # "Normal"
                  }
                  frame 3001..3600 {
                  }
                  frame 3601.. {
                  }
                }
                n2782 = Or(x=w4136, y=w4135) -> (x .or. y?=w4134:bool)
                n2783 = Greater Or Equal?(x=w4139, y=w4123) -> (x >= y?=w4126:bool)
                n2784 = case shown="0, 1, Default" w4139 {
                  tunnel: [1 3] -> w4122
                  frame 0, 1, Default {
                  }
                  frame 2.. {
                  }
                }
                n2785 = case shown="True" w4126 {
                  tunnel: [1 3] -> w4121
                  frame False {
                  }
                  frame True {
                  }
                }
                n2786 = case shown="True" w4134 {
                  tunnel: [1 2] -> w4120
                  frame False {
                  }
                  frame True {
                  }
                }
                n2787 = Build Array(w4146, w4145, w4144) -> (w4143:i32[])
                n2788 = Number To Decimal String(number=w4158) -> (decimal integer string=→"sp_st":string)  [unwired: 1 in]
                n2789 = Array Max & Min(array=w4143) -> (max value=w4140:i32)  [unwired: 3 out]
                "TEMP STATE" <- w4140
                n2790 = Number To Decimal String(number=w4164) -> (decimal integer string=w4167:string)  [unwired: 1 in]
                n2791 = Number To Decimal String(number=w4163) -> (decimal integer string=w4165:string)  [unwired: 1 in]
                n2792 = Number To Decimal String(number=w4140) -> (decimal integer string=→"temp_st":string)  [unwired: 1 in]
                n2793 = Build Array(w4122, w4121, w4120) -> (w4119:i32[])
                n2794 = local write "nl_st"(w4167) -> ()
                n2795 = local write "ff_st"(w4165) -> ()
                n2796 = Number To Decimal String(number=1) -> (decimal integer string=w4162:string)  [unwired: 1 in]
                n2797 = Array Max & Min(array=w4119) -> (max value=w4118:i32)  [unwired: 3 out]
                n2798 = local write "Air temp"(w4162) -> ()
                n2799 = Number To Decimal String(number=w4118) -> (decimal integer string=w4117:string)  [unwired: 1 in]
                n2800 = local write "Stroke Ln 2"(w4117) -> ()
              }
            }
            n2801 = local read "Stroke Ln 2"() -> (w4029:string)
            n2802 = local read "nl_st"() -> (w4035:string)
            n2803 = local read "ff_st"() -> (w4032:string)
            n2804 = local read "sp_st"() -> (w4033:string)
            n2805 = local read "temp_st"() -> (w4034:string)
            n2806 = local read "Air temp"() -> (w4028:string)
            n2807 = Replace Array Subset(array="in", new element #1=w4035, index #1=1 ("index"), new element #2=w4032, index #2=2 ("index"), new element #3=w4034, index #3=3 ("index"), new element #4=w4033, index #4=4 ("index"), new element #5=w4029, index #5=5 ("index"), new element #6=w4028, index #6=6 ("index"), new element #7="Sensor State" ("new element/subarray"), index #7=0 ("index")) -> (→"out":string[])
          }
        }
        n2808 = Wait (ms)(milliseconds to wait=u32 10) -> ()  [unwired: 1 out]
        n2809 = local read "EXIT"() -> (w4024:bool)
      }
      n2810 = while {
        stop <- w3998 stop-if-true
        n2811 = local read "run replace"() -> (w4000:bool)
        n2812 = Wait (ms)(milliseconds to wait=u32 100) -> ()  [unwired: 1 out]
        n2813 = Equal?(x="FLAG 2", y=0.0) -> (x = y?=w4001:bool)
        n2814 = case shown="True" w4001 {
          frame False {
          }
          frame True {
            n2815 = local write "FLAG 2"(100.0 ("FLAG 2")) -> ()
            n2816 = call <vilib>:"Read Characters From File.vi"("file path (dialog if empty)"=path "C:/LAB-IQ-NXT/WO 2449 TT.sig", "convert eol? (no:F)"=FALSE ("append to file? (new file:F)")) -> ("character string"=w4004:string)  [unwired: 4 in, 3 out]
            n2817 = call <vilib>:"Read Characters From File.vi"("file path (dialog if empty)"=path "C:/LAB-IQ-NXT/WO 2449 TRH.sig", "convert eol? (no:F)"=FALSE ("append to file? (new file:F)")) -> ("character string"=w4005:string)  [unwired: 4 in, 3 out]
            n2818 = Decimal String To Number(string=w4004) -> (number=w4006:i32)  [unwired: 2 in, 1 out]
            n2819 = local write "Total No. of Tests"(w4006) -> ()
            n2820 = Decimal String To Number(string=w4005) -> (number=w4009:i32)  [unwired: 2 in, 1 out]
            n2821 = local write "SEN.RUN HRS"(w4009) -> ()
          }
        }
        n2822 = case shown="True" w4000 {
          frame False {
          }
          frame True {
            n2823 = Equal?(x="FLAG 4", y=0.0) -> (x = y?=w4013:bool)
            n2824 = case shown="False" w4013 {
              frame False {
                n2825 = Get Date/Time In Seconds() -> (seconds since 1Jan1904=w4019:timestamp)
                n2826 = local read "START 3"() -> (w4017:dbl)
                n2827 = To Double Precision Float(number=w4019) -> (double precision float=w4018:dbl)
                n2828 = Subtract(x=w4018, y=w4017) -> (x-y=→"SENSOR TIME":dbl)
              }
              frame True {
                n2829 = Get Date/Time In Seconds() -> (seconds since 1Jan1904=w4021:timestamp)
                n2830 = local write "FLAG 4"(100.0 ("FLAG")) -> ()
                n2831 = To Double Precision Float(number=w4021) -> (double precision float=→"START 3":dbl)
              }
            }
          }
        }
        n2832 = local read "EXIT"() -> (w3998:bool)
      }
      n2833 = while {
        shift-right: [w3796] -> _
        shift-left: _ -> [w3797]
        tunnel: [w3791] -> _
        i -> [w3791]
        stop <- w3790 stop-if-true
        n2834 = Wait (ms)(milliseconds to wait=u32 50 ("Refresh Rate (ms)")) -> ()  [unwired: 1 out]
        n2835 = local read "Json End Flg"() -> (w3792:bool)
        n2836 = Not(x="Upld AR 2") -> ()  [unwired: 1 out]
        n2837 = local read "Upld AR 2"() -> (w3793:bool)
        n2838 = call "Elapsed Time9"("Time Target (s)"="Sen.Upload Rate (s)", "Reset"=FALSE, "Auto Reset"=TRUE) -> ("Time has Elapsed"=w3803:bool)  [unwired: 9 in, 7 out]
        n2839 = Or(x=w3803, y=w3792) -> (x .or. y?=w3799:bool)
        n2840 = case shown="True" w3799 {
          frame False {
          }
          frame True {
            w3897 = "\"SensorName\":\"" ("string")
            w3867 = " \"},{"
            w3892 = "\",\"SensorState\":\""
            w3894 = "\",\"SensorModelNumber\":\"" ("string")
            w3893 = "\",\"SensorRuntimeHours\":\"" ("string")
            n2841 = local read "model num"() -> (w3891:string[])
            n2842 = local read "Sensor name"() -> (w3910:string[])
            n2843 = local read "run"() -> (w3881:string[])
            n2844 = local read "SENSOR TIME"() -> (w3836:dbl)
            n2845 = local read "out"() -> (w3829:string[])
            n2846 = local read "Total No. of Tests"() -> (w3834:dbl)
            n2847 = Select(t=60.0, s="Run test 3", f=3600.0) -> (s? t:f=w3845:dbl)
            n2848 = Index Array(array=w3891, index #1=1 ("index")) -> (element #1=w3890:string, element #2=w3889:string, element #3=w3888:string, element #4=w3887:string, element #5=w3886:string, element #6=w3885:string)  [unwired: 5 in]
            n2849 = Index Array(array=w3881, index #1=1 ("index")) -> (element #1=w3880:string, element #2=w3879:string, element #3=w3878:string, element #4=w3877:string, element #5=w3876:string, element #6=w3875:string)  [unwired: 5 in]
            n2850 = Index Array(array=w3910, index #1=1 ("index")) -> (element #1=w3909:string, element #2=w3908:string, element #3=w3907:string, element #4=w3906:string, element #5=w3896:string, element #6=w3895:string)  [unwired: 5 in]
            n2851 = Index Array(array=w3829, index #1=1 ("index")) -> (element #1=w3862:string, element #2=w3861:string, element #3=w3860:string, element #4=w3859:string, element #5=w3858:string, element #6=w3857:string)  [unwired: 5 in]
            n2852 = local read "SEN.RUN HRS"() -> (w3832:dbl)
            n2853 = Divide(x=w3836, y=w3845) -> (x/y=w3844:dbl)
            n2854 = Increment(x=w3844) -> (x+1=w3839:dbl)
            n2855 = Number To Decimal String(number=w3839) -> (decimal integer string=→"run hrs":string)  [unwired: 1 in]
            n2856 = Divide(x=w3832, y=3600.0 ("f")) -> (x/y=w3827:dbl)
            n2857 = Round To Nearest(number=w3827) -> (nearest integer value=w3825:dbl)
            n2858 = Number To Decimal String(number=w3825) -> (decimal integer string=w3826:string)  [unwired: 1 in]
            n2859 = Number To Decimal String(number=w3834) -> (decimal integer string=w3835:string)  [unwired: 1 in]
            n2860 = local read "Model No"() -> (w3840:string)
            n2861 = local read "UUID"() -> (w3936:string)
            n2862 = local read "Serial No"() -> (w3940:string)
            n2863 = local read "Secret Key"() -> (w3941:string)
            n2864 = Concatenate Strings("\",\"MachineSerialNumber\":\"" ("string"), w3940) -> (w3944:string)
            n2865 = Concatenate Strings("\",\"ModelNumber\":\"" ("string"), w3840) -> (w3841:string)
            n2866 = Concatenate Strings("\",\"MachineRuntimeHours\":\"" ("string"), w3826) -> (w3945:string)
            n2867 = Concatenate Strings("\",\"MachineRuntimeCycles\":\"", w3835) -> (w3938:string)
            n2868 = Concatenate Strings(w3894, w3890) -> (w3924:string)
            n2869 = Concatenate Strings(w3893, w3880) -> (w3925:string)
            n2870 = Concatenate Strings(w3892, w3862) -> (w3923:string)
            n2871 = Concatenate Strings(w3944, w3841, w3945, w3938) -> (w3947:string)
            n2872 = Concatenate Strings(w3894, w3889) -> (w3921:string)
            n2873 = Concatenate Strings(w3893, w3879) -> (w3920:string)
            n2874 = Concatenate Strings(w3892, w3861) -> (w3922:string)
            n2875 = Concatenate Strings(w3894, w3888) -> (w3916:string)
            n2876 = Concatenate Strings(w3893, w3878) -> (w3917:string)
            n2877 = Concatenate Strings(w3892, w3860) -> (w3915:string)
            n2878 = Concatenate Strings(w3894, w3887) -> (w3913:string)
            n2879 = Concatenate Strings(w3893, w3877) -> (w3912:string)
            n2880 = Concatenate Strings(w3892, w3859) -> (w3914:string)
            n2881 = Concatenate Strings(w3924, w3925, w3923) -> (w3926:string)
            n2882 = Concatenate Strings(w3894, w3886) -> (w3903:string)
            n2883 = Concatenate Strings(w3893, w3876) -> (w3904:string)
            n2884 = Concatenate Strings(w3894, w3885) -> (w3900:string)
            n2885 = Concatenate Strings(w3893, w3875) -> (w3899:string)
            n2886 = Concatenate Strings(w3892, w3858) -> (w3902:string)
            n2887 = Concatenate Strings(w3892, w3857) -> (w3901:string)
            n2888 = Concatenate Strings("{\"SecretKey\":\"", w3941, w3947, "\",\"UUID\" : \"", w3936, "\",\"SensorInformation\":", "[{" ("string")) -> (w3874:string)
            n2889 = Concatenate Strings(w3921, w3920, w3922) -> (w3919:string)
            n2890 = Concatenate Strings(w3916, w3917, w3915) -> (w3918:string)
            n2891 = Concatenate Strings(w3913, w3912, w3914) -> (w3911:string)
            n2892 = Concatenate Strings(w3903, w3904, w3902) -> (w3905:string)
            n2893 = Concatenate Strings(w3900, w3899, w3901) -> (w3898:string)
            n2894 = Concatenate Strings(w3897, w3909, w3926, w3867) -> (w3873:string)
            n2895 = Concatenate Strings(w3897, w3908, w3919, w3867) -> (w3872:string)
            n2896 = Concatenate Strings(w3897, w3907, w3918, w3867) -> (w3871:string)
